vi "SetAngleDecel.vi"(0 "Time Manager Output":dbl, 1 "ta > tf/2?":bool, 5 "Angular Velocity":dbl, 7 "Angular Acceleration":dbl, 9 "Time Acceleration":dbl, 11 "Time Cruise":dbl, 12 "Time Finished":dbl) -> (8 "CurrentAngle":dbl)   [LabVIEW 2015]
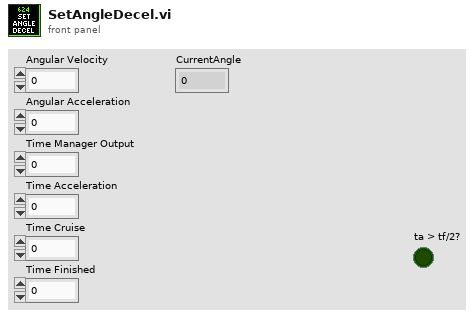
[diagram p1: front panel]
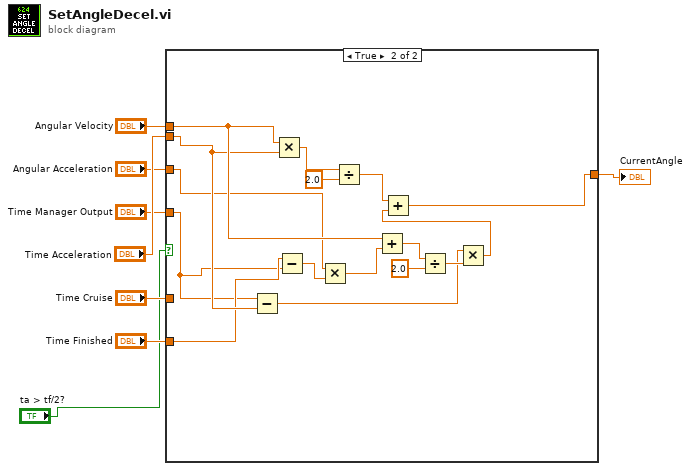
[diagram p0: block diagram]
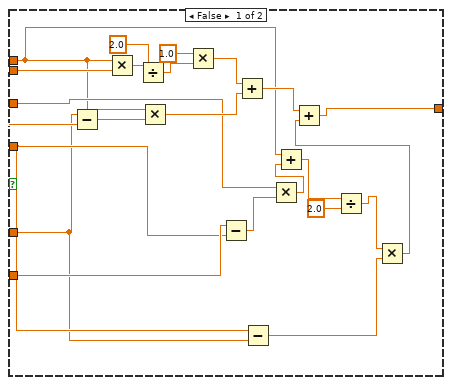
[diagram p2: hidden frame]
diagram:
  n1 = case shown="True" "ta > tf/2?" {
    tunnel: "Time Acceleration" -> [w28 w42]
    tunnel: "Time Finished" -> [w21 w40]
    tunnel: "Angular Acceleration" -> [w19 w41]
    tunnel: "Angular Velocity" -> [w18 w43]
    tunnel: "Time Manager Output" -> [w14 w39]
    tunnel: "Time Cruise" -> [w13 _]
    tunnel: [w9 w31] -> w2
    frame False {
      n2 = Subtract(x=w13, y=w28) -> (x-y=w27:dbl)
      n3 = Multiply(x=w18, y=w28) -> (x*y=w30:dbl)
      n4 = Divide(x=w30, y=2.0) -> (x/y=w26:dbl)
      n5 = Multiply(x=w18, y=w27) -> (x*y=w24:dbl)
      n6 = Multiply(x=1.0, y=w26) -> (x*y=w23:dbl)
      n7 = Subtract(x=w21, y=w14) -> (x-y=w20:dbl)
      n8 = Add(x=w23, y=w24) -> (x+y=w22:dbl)
      n9 = Subtract(x=w14, y=w13) -> (x-y=w12:dbl)
      n10 = Multiply(x=w19, y=w20) -> (x*y=w17:dbl)
      n11 = Add(x=w18, y=w17) -> (x+y=w16:dbl)
      n12 = Divide(x=w16, y=2.0) -> (x/y=w11:dbl)
      n13 = Multiply(x=w11, y=w12) -> (x*y=w10:dbl)
      n14 = Add(x=w22, y=w10) -> (x+y=w9:dbl)
    }
    frame True {
      n15 = Subtract(x=w39, y=w42) -> (x-y=w33:dbl)
      n16 = Multiply(x=w43, y=w42) -> (x*y=w46:dbl)
      n17 = Subtract(x=w40, y=w39) -> (x-y=w38:dbl)
      n18 = Multiply(x=w41, y=w38) -> (x*y=w37:dbl)
      n19 = Divide(x=w46, y=2.0) -> (x/y=w44:dbl)
      n20 = Add(x=w43, y=w37) -> (x+y=w36:dbl)
      n21 = Divide(x=w36, y=2.0) -> (x/y=w34:dbl)
      n22 = Multiply(x=w33, y=w34) -> (x*y=w32:dbl)
      n23 = Add(x=w44, y=w32) -> (x+y=w31:dbl)
    }
  }
  "CurrentAngle" <- w2
